vi "mono_send_gps_config.vi"(0 "GPS Configuration Path":path=path "C:/Users/celit/Documents/GitHub/client/configurations/camera/demo_camera.json", 1 "simulator ip":string, 2 "TCP Network Connection in":refnum<k5>, 3 "error in":errorcluster) -> (5 "config response":string, 6 "sensor connection ID":refnum<k5>, 7 "TCP Network Connection out":refnum<k5>, 8 "error out":errorcluster)   [LabVIEW 2018, in "monoDrive.lvlib"]
uses:
  monoDrive.lvlib
  mono_commands.ctl
panel:
  in  "sensor":T1
  out "stream response":string
  in  "vehicle_id":string="1"
  out "JSON string 2":string
  out "error out 3":errorcluster
  out "text":string
  out "JSON string":string
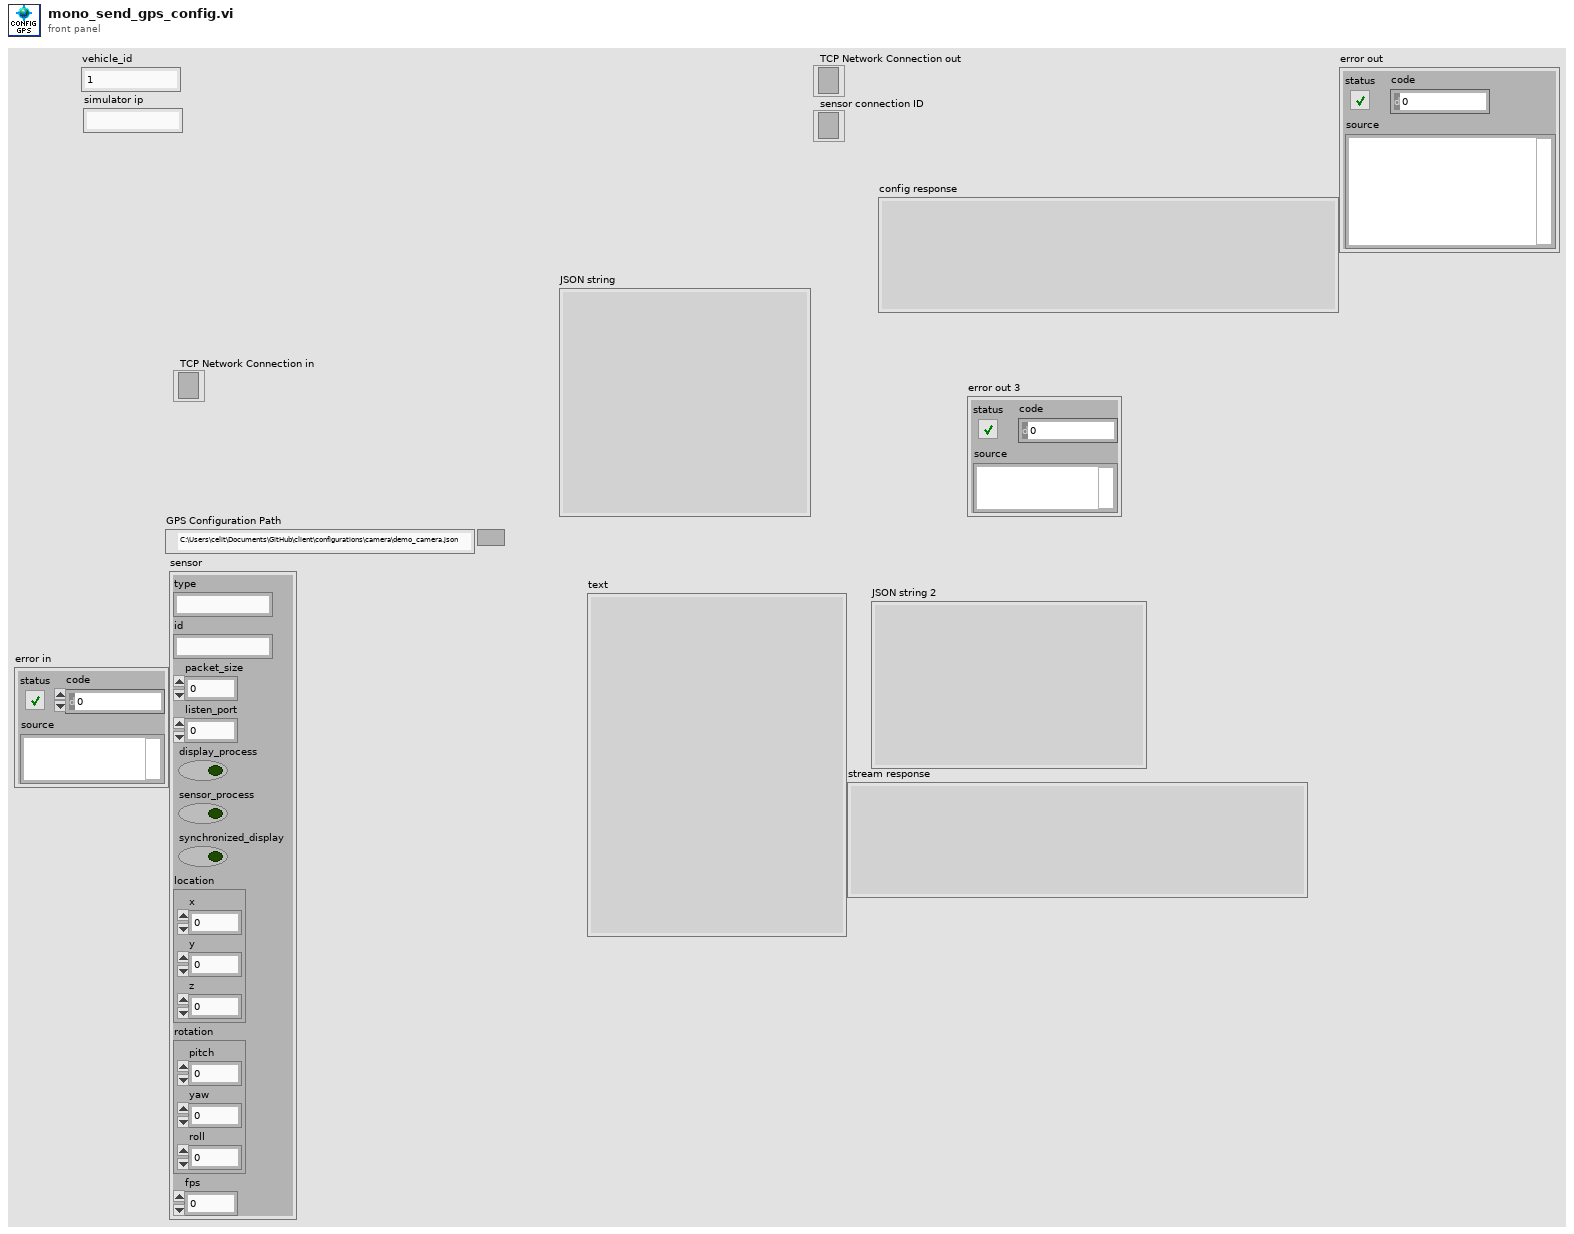
[diagram p1: front panel]
types:
  T1 = cluster{"type":string, "id":string, "packet_size":i32, "listen_port":i32, "display_process":bool, "sensor_process":bool, "synchronized_display":bool, "location":cluster{"x":i32, "y":i32, "z":i32}, "rotation":cluster{"pitch":i32, "yaw":i32, "roll":i32}, "fps":i32}
  T2 = cluster{"type":string, "success":bool, "reference":i32, "message":cluster{"vehicle_id":string, "sensor":cluster{"type":string, "id":string, "packet_size":i32, "listen_port":i32, "display_process":bool, "sensor_process":bool, "synchronized_display":bool, "location":cluster{"x":i32, "y":i32, "z":i32}, "rotation":cluster{"pitch":i32, "yaw":i32, "roll":i32}, "fps":i32}}}
  T3 = cluster{"vehicle_id":string, "sensor":cluster{"type":string, "id":string, "packet_size":i32, "listen_port":i32, "display_process":bool, "sensor_process":bool, "synchronized_display":bool, "location":cluster{"x":i32, "y":i32, "z":i32}, "rotation":cluster{"pitch":i32, "yaw":i32, "roll":i32}, "fps":i32}}
  T4 = typedef "monoDrive.lvlib/mono_commands.ctl" = cluster{"SIMULATOR_STATUS_UUID":string, "STREAM_DATA_COMMAND_UUID":string, "SIMULATOR_CONFIG_COMMAND_UUID":string, "VEHICLE_CONFIG_COMMAND_UUID":string, "EGO_CONTROL_COMMAND_UID":string, "WAYPOINT_UPDATE_COMMAND_UID":string, "SCENARIO_COMMAND_UID":string, "MAP_COMMAND_UID":string, "SPAWN_COMMAND_UID":string, "MOVE_ACTOR_COMMAND_UID":string, "SCENARIO_INIT_COMMAND_UID":string, "ATTACH_SENSOR_COMMAND_UID":string, "DETACH_SENSOR_COMMAND_UID":string, "CONTROL_HEADER":string, "RESPONSE_HEADER":string}
  T5 = cluster{"type":string, "id":string, "packet_size":i32, "listen_port":i32}
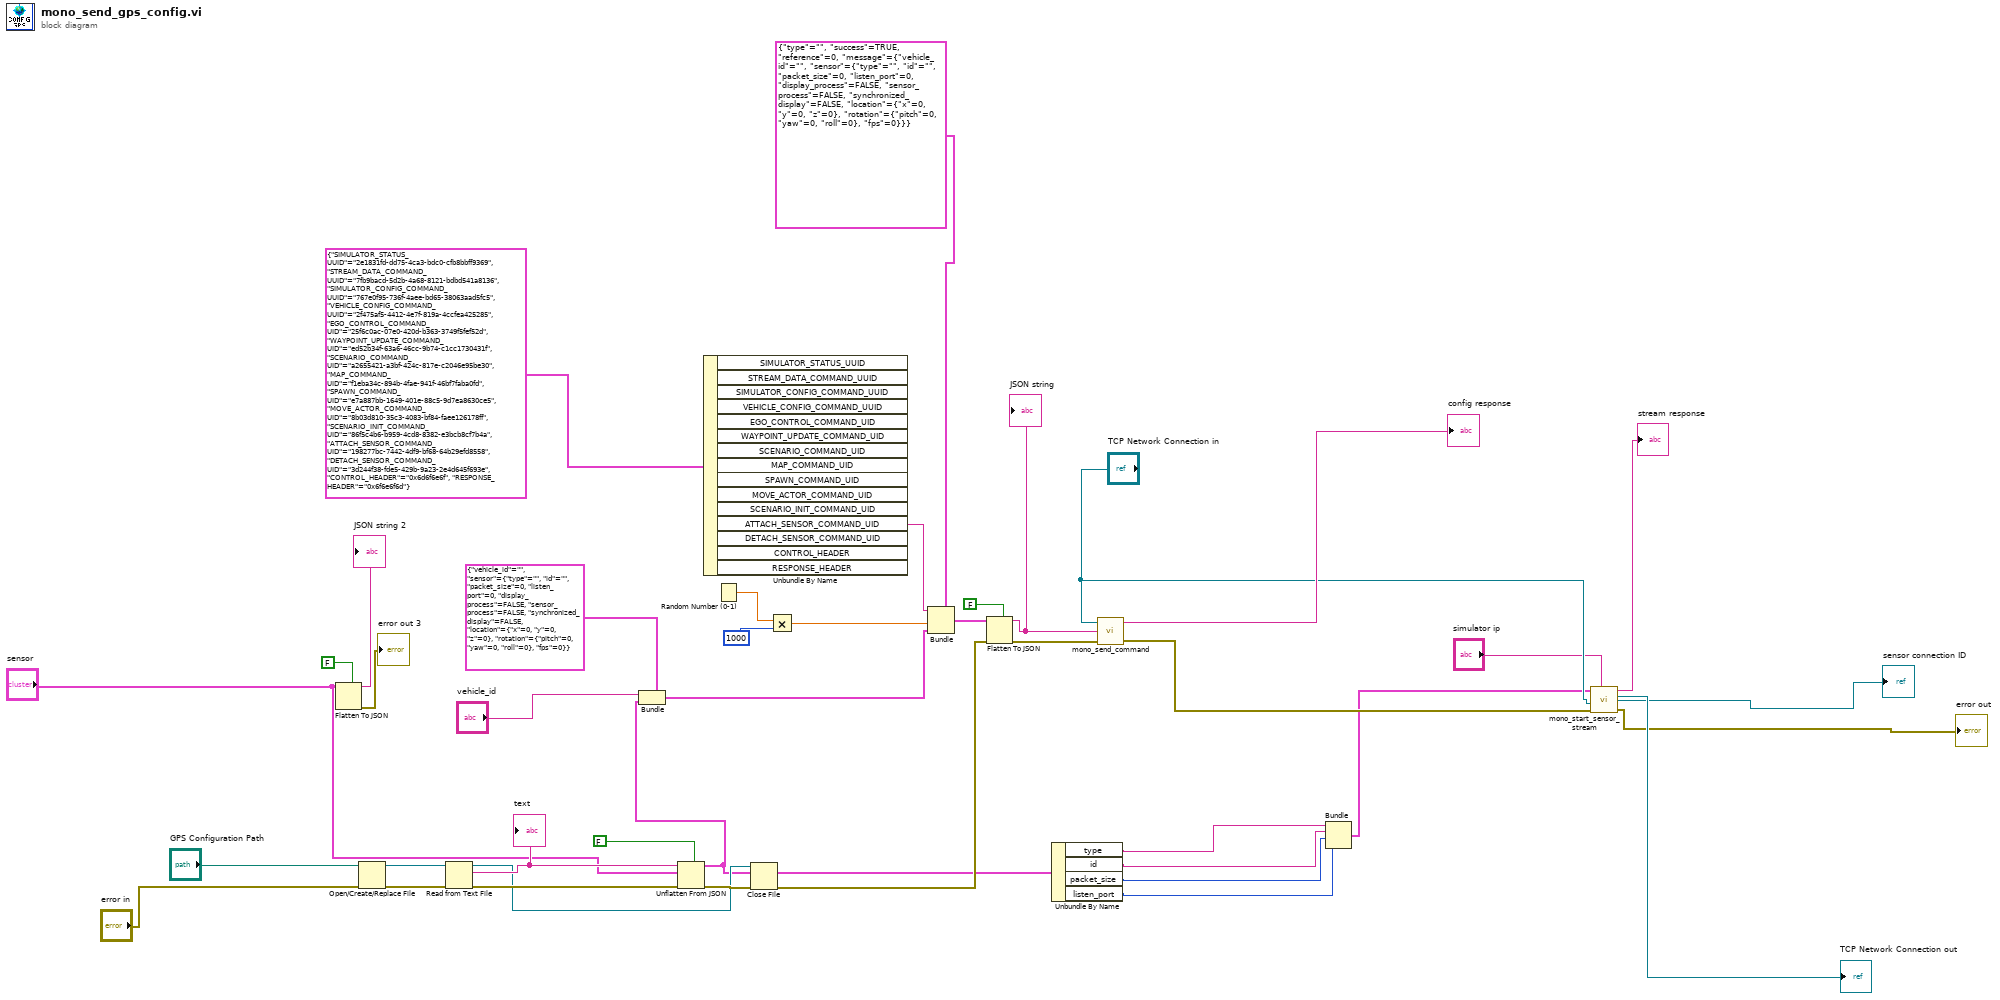
[diagram p0: block diagram]
diagram:
  n1 = Flatten To JSON(enable LabVIEW extensions? (T)=FALSE, anything="sensor") -> (JSON string=→"JSON string 2":string, 11:→"error out 3":errorcluster)  [unwired: 1 in]
  n2 = Open/Create/Replace File(file path (use dialog)="GPS Configuration Path", error in="error in") -> (refnum out=w30:refnum<file>, error out=w32:errorcluster)  [unwired: 4 in, 1 out]
  n3 = Read from Text File(file (use dialog)=w30, error in=w32) -> (refnum out=w28:refnum<file>, text=w34:string, error out=w35:errorcluster)  [unwired: 2 in, 1 out]
  "text" <- w34
  n4 = Unflatten From JSON(enable LabVIEW extensions? (T)=FALSE, JSON string=w34, type and defaults="sensor", error in (no error)=w35) -> (value=w1:T1, error out=w36:errorcluster)  [unwired: 3 in]
  n5 = Bundle(cluster=T3 {"vehicle_id"="", "sensor"={"type"="", "id"="", "packet_size"=0, "listen_port"=0, "display_process"=FALSE, "sensor_process"=FALSE, "synchronized_display"=FALSE, "location"={"x"=0, "y"=0, "z"=0}, "rotation"={"pitch"=0, "yaw"=0, "roll"=0}, "fps"=0}}, "vehicle_id"="vehicle_id", "sensor"=w1) -> (w2:T3)
  n6 = Unbundle By Name(T4 {"SIMULATOR_STATUS_UUID"="2e1831fd-dd75-4ca3-bdc0-cfb8bbff9369", "STREAM_DATA_COMMAND_UUID"="7fb9bacd-5d2b-4a68-8121-bdbd541a8136", "SIMULATOR_CONFIG_COMMAND_UUID"="767e0f95-736f-4aee-bd65-38063aad5fc5", "VEHICLE_CONFIG_COMMAND_UUID"="2f475af5-4412-4e7f-819a-4ccfea425285", "EGO_CONTROL_COMMAND_UID"="25f6c0ac-07e0-420d-b363-3749f5fef52d", "WAYPOINT_UPDATE_COMMAND_UID"="ed52b34f-63a6-46cc-9b74-c1cc1730431f", "SCENARIO_COMMAND_UID"="a2655421-a3bf-424c-817e-c2046e95be30", "MAP_COMMAND_UID"="f1eba34c-894b-4fae-941f-46bf7faba0fd", "SPAWN_COMMAND_UID"="e7a887bb-1649-401e-88c5-9d7ea8630ce5", "MOVE_ACTOR_COMMAND_UID"="8b03d810-35c3-4083-bf84-faee126178ff", "SCENARIO_INIT_COMMAND_UID"="86f5c4b6-b959-4cd8-8382-e3bcb8cf7b4a", "ATTACH_SENSOR_COMMAND_UID"="198277bc-7442-4df9-bf68-64b29efd8558", "DETACH_SENSOR_COMMAND_UID"="3d244f38-fde5-429b-9a23-2e4d645f693e", "CONTROL_HEADER"="0x6d6f6e6f", "RESPONSE_HEADER"="0x6f6e6f6d"} ("Cluster")) -> ("ATTACH_SENSOR_COMMAND_UID"=w37:string)  [unwired: 14 out]
  n7 = Random Number (0-1)() -> (number: 0 to 1=w11:dbl)
  n8 = Close File(refnum=w28, error in=w36) -> (error out=w29:errorcluster)  [unwired: 1 out]
  n9 = Multiply(x=w11, y=1000) -> (x*y=w8:dbl)
  n10 = Bundle(cluster=T2 {"type"="", "success"=TRUE, "reference"=0, "message"={"vehicle_id"="", "sensor"={"type"="", "id"="", "packet_size"=0, "listen_port"=0, "display_process"=FALSE, "sensor_process"=FALSE, "synchronized_display"=FALSE, "location"={"x"=0, "y"=0, "z"=0}, "rotation"={"pitch"=0, "yaw"=0, "roll"=0}, "fps"=0}}}, "type"=w37, "reference"=w8, "message"=w2) -> (w27:T2)  [unwired: 1 in]
  n11 = Flatten To JSON(enable LabVIEW extensions? (T)=FALSE, anything=w27, error in (no error)=w29) -> (JSON string=w38:string, 11:w41:errorcluster)
  "JSON string" <- w38
  n12 = Unbundle By Name(w1) -> ("type"=w6:string, "id"=w5:string, "packet_size"=w4:i32, "listen_port"=w3:i32)
  n13 = call "mono_send_command.vi"("error in (no error)"=w41, "JSON Command"=w38, "TCP Network Connection in"="TCP Network Connection in") -> ("error out"=w19:errorcluster, "response"=→"config response":string)  [unwired: 1 in]
  n14 = Bundle("type"=w6, "id"=w5, "packet_size"=w4, "listen_port"=w3) -> (w15:T5)  [unwired: 1 in]
  n15 = call "mono_start_sensor_stream.vi"("input cluster"=w15, "TCP Network Connection in"="TCP Network Connection in", "error in"=w19, "simulator ip"="simulator ip") -> ("TCP Network Connection out"=→"TCP Network Connection out":refnum<k5>, "stream response"=→"stream response":string, "sensor connection ID"=→"sensor connection ID":refnum<k5>, "error out"=→"error out":errorcluster)
